vi "06 LV - Video Lifecycle.vi"() -> ()   [LabVIEW 2020]
uses:
  client/Video/Video.lvclass/Video.ctl
  client/Video/Video.lvclass
  client/Client/Client.lvclass
  client/VideoCreateStaging/VideoCreateStaging.lvclass
  client/List/List.lvclass
panel:
  out "video created found":bool
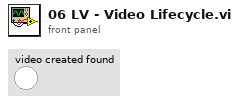
[diagram p1: front panel]
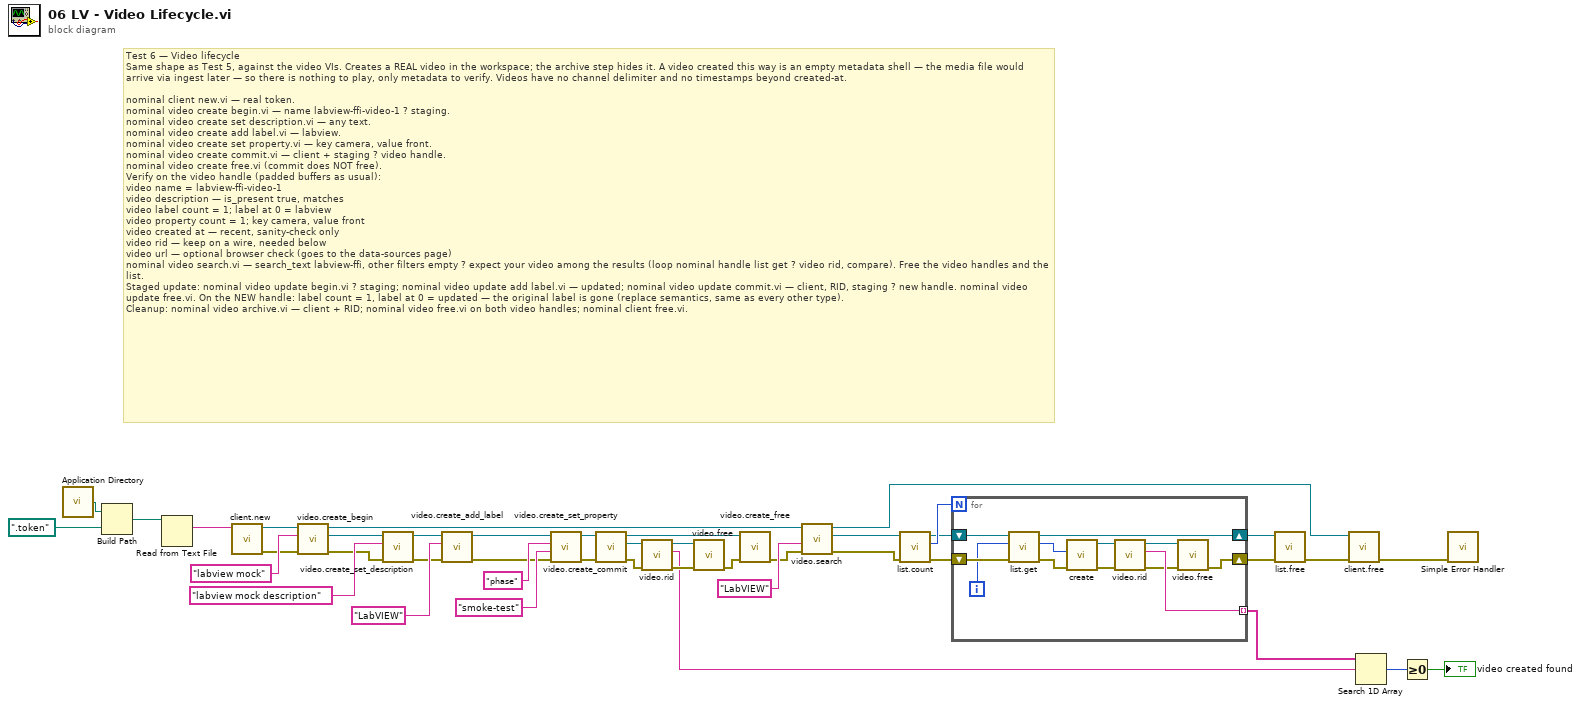
[diagram p0: block diagram]
diagram:
  # "Test 6 — Video lifecycle\nSame shape as Test 5, against the video VIs. Creates a REAL video in the workspace; the archive step hides it. A video created this way is an empty metadata shell — the media file would arrive via ingest later — so there is nothing to play, only metadata to verify. Videos have no channel delimiter and no timestamps beyond created-at.\n\nnominal client new.vi — real token.\nnominal video create begin.vi — name labview-ffi-video-1 ? staging.\nnominal video create set description.vi — any text.\nnominal video create add label.vi — labview.\nnominal video create set property.vi — key camera, value front.\nnominal video create commit.vi — client + staging ? video handle.\nnominal video create free.vi (commit does NOT free).\nVerify on the video handle (padded buffers as usual):\nvideo name = labview-ffi-video-1\nvideo description — is_present true, matches\nvideo label count = 1; label at 0 = labview\nvideo property count = 1; key camera, value front\nvideo created at — recent, sanity-check only\nvideo rid — keep on a wire, needed below\nvideo url — optional browser check (goes to the data-sources page)\nnominal video search.vi — search_text labview-ffi, other filters empty ? expect your video among the results (loop nominal handle list get ? video rid, compare). Free the video handles and the list.\nStaged update: nominal video update begin.vi ? staging; nominal video update add label.vi — updated; nominal video update commit.vi — client, RID, staging ? new handle. nominal video update free.vi. On the NEW handle: label count = 1, label at 0 = updated — the original label is gone (replace semantics, same as every other type).\nCleanup: nominal video archive.vi — client + RID; nominal video free.vi on both video handles; nominal client free.vi."
  n1 = call <vilib>:"Application Directory.vi"() -> ("Application Directory"=w42:path)
  n2 = Build Path(base path=w42, name or relative path=path ".token") -> (appended path=w40:path)
  n3 = Read from Text File(file (use dialog)=w40) -> (text=w36:string)  [unwired: 3 in, 3 out]
  n4 = call "client.new.vi"("token"=w36) -> ("error out"=w33:errorcluster, "Client out"=w34:refnum<class "Client.lvclass">)  [unwired: 9 in]
  n5 = call "video.create_begin.vi"("error in"=w33, "name"="labview mock", "Client in"=w34) -> ("error out"=w30:errorcluster, "VideoCreateStaging"=w31:refnum<class "VideoCreateStaging.lvclass">, "Client out"=w11:refnum<class "Client.lvclass">)  [unwired: 6 in]
  n6 = call "video.create_set_description.vi"("error in"=w30, "description"="labview mock description" ("name"), "VideoCreateStaging in"=w31) -> ("error out"=w28:errorcluster, "VideoCreateStaging out"=w27:refnum<class "VideoCreateStaging.lvclass">)  [unwired: 7 in]
  n7 = call "video.create_add_label.vi"("error in"=w28, "label"="LabVIEW" ("name"), "VideoCreateStaging in"=w27) -> ("error out"=w23:errorcluster, "VideoCreateStaging out"=w24:refnum<class "VideoCreateStaging.lvclass">)  [unwired: 7 in]
  n8 = call "video.create_set_property.vi"("error in"=w23, "value"="smoke-test" ("name"), "key"="phase" ("name"), "VideoCreateStaging in"=w24) -> ("error out"=w21:errorcluster, "VideoCreateStaging out"=w22:refnum<class "VideoCreateStaging.lvclass">)  [unwired: 6 in]
  n9 = call "video.create_commit.vi"("error in"=w21, "VideoCreateStaging in"=w22) -> ("error out"=w14:errorcluster, "Video"=w19:refnum<class "Video.lvclass">, "VideoCreateStaging out"=w20:refnum<class "VideoCreateStaging.lvclass">)  [unwired: 7 in]
  n10 = call "video.rid.vi"("error in"=w14, "Video in"=w19) -> ("error out"=w17:errorcluster, "rid"=w16:string, "Video out"=w18:refnum<class "Video.lvclass">)  [unwired: 7 in]
  n11 = call "video.free.vi"("error in"=w17, "Video"=w18) -> ("error out"=w15:errorcluster)  [unwired: 9 in]
  n12 = call "video.create_free.vi"("error in"=w15, "VideoCreateStaging"=w20) -> ("error out"=w12:errorcluster)  [unwired: 9 in]
  n13 = call "video.search.vi"("error in"=w12, "label"="LabVIEW", "Client in"=w11) -> ("error out"=w2:errorcluster, "List"=w1:refnum<class "List.lvclass">, "Client out"=w6:refnum<class "Client.lvclass">)  [unwired: 6 in]
  n14 = call "list.count.vi"("error in"=w2, "List in"=w1) -> ("error out"=w3:errorcluster, "count"=w5:u32, "List out"=w4:refnum<class "List.lvclass">)  [unwired: 7 in]
  n15 = for {
    N: w5 -> [_]
    shift-right: [w46] -> w9
    shift-left: w3 -> [w51]
    tunnel: [w47] -> w39 mode=indexing
    shift-right: [w43] -> w10
    shift-left: w4 -> [w49]
    i -> [w50]
    n16 = call "list.get.vi"("error in"=w51, "index"=w50, "List in"=w49) -> ("error out"=w52:errorcluster, "handle"=w54:i32, "List out"=w43:refnum<class "List.lvclass">)  [unwired: 6 in]
    n17 = call "create.vi"("error in (no error)"=w52, "handle"=w54) -> ("error out"=w44:errorcluster, "Video"=w53:refnum<class "Video.lvclass">)  [unwired: 8 in]
    n18 = call "video.rid.vi"("error in"=w44, "Video in"=w53) -> ("error out"=w45:errorcluster, "rid"=w47:string, "Video out"=w48:refnum<class "Video.lvclass">)  [unwired: 7 in]
    n19 = call "video.free.vi"("error in"=w45, "Video"=w48) -> ("error out"=w46:errorcluster)  [unwired: 9 in]
  }
  n20 = call "list.free.vi"("error in"=w9, "List in"=w10) -> ("error out"=w8:errorcluster)  [unwired: 9 in]
  n21 = call "client.free.vi"("error in"=w8, "Client in"=w6) -> ("error out"=w7:errorcluster)  [unwired: 9 in]
  n22 = Search 1D Array(1D array=w39, element=w16) -> (index of element=w38:i32)  [unwired: 1 in]
  n23 = Greater Or Equal To 0?(x=w38) -> (x >= 0?=→"video created found":bool)
  n24 = call <vilib>:"Simple Error Handler.vi"("error in (no error)"=w7) -> ()  [unwired: 4 in, 5 out]
